vi "Get 2D Array Double.vi"(5 "use temporary file? (F)":bool, 7 "data type of variable":dbl[][](array[numeric]), 8 "error in":errorcluster, 10 "variable name":string, 11 "GOLPI ref. in":T1={"pipe handle"={"lv_proc.dll file path"=path "", "process instance handle"=[], "debug mode"=FALSE, "debug data"=[]}, "fast read timeout [ms]"=500, "fast read settle time [ms]"=10, "fast read to multiple [ms]"=1, "max elements per input line"=100, "slow read timeout [ms]"=5000, "stdin double format specifier"="%_16e", "max elements per stdout output column"=100, "console mode bitstream"=FALSE, "bitstream first read timeout [ms]"=1000, "bitstream read timeout [ms]"=50, "struct transfer possible"=FALSE, "matlab mode"=FALSE}) -> (0 "error out":errorcluster, 2 "value":dbl[][](array[numeric]) format="%.2f", 3 "GOLPI ref. out":T1={"pipe handle"={"lv_proc.dll file path"=path "", "process instance handle"=[], "debug mode"=FALSE, "debug data"=[]}, "fast read timeout [ms]"=500, "fast read settle time [ms]"=10, "fast read to multiple [ms]"=1, "max elements per input line"=100, "slow read timeout [ms]"=5000, "stdin double format specifier"="%_16e", "max elements per stdout output column"=100, "console mode bitstream"=FALSE, "bitstream first read timeout [ms]"=1000, "bitstream read timeout [ms]"=50, "struct transfer possible"=FALSE, "matlab mode"=FALSE})   [LabVIEW 2020, in "GOLPI library.lvlib"]
doc: "Part of polymorph Get Variable.vi"
uses:
  GOLPI library.lvlib
  GOLPI reference Type Def.ctl
  Pipe Handle.ctl
  Bitstream Data Type.ctl
  Custom Error Codes Enum Type Def.vi
  LV Process library.lvlib
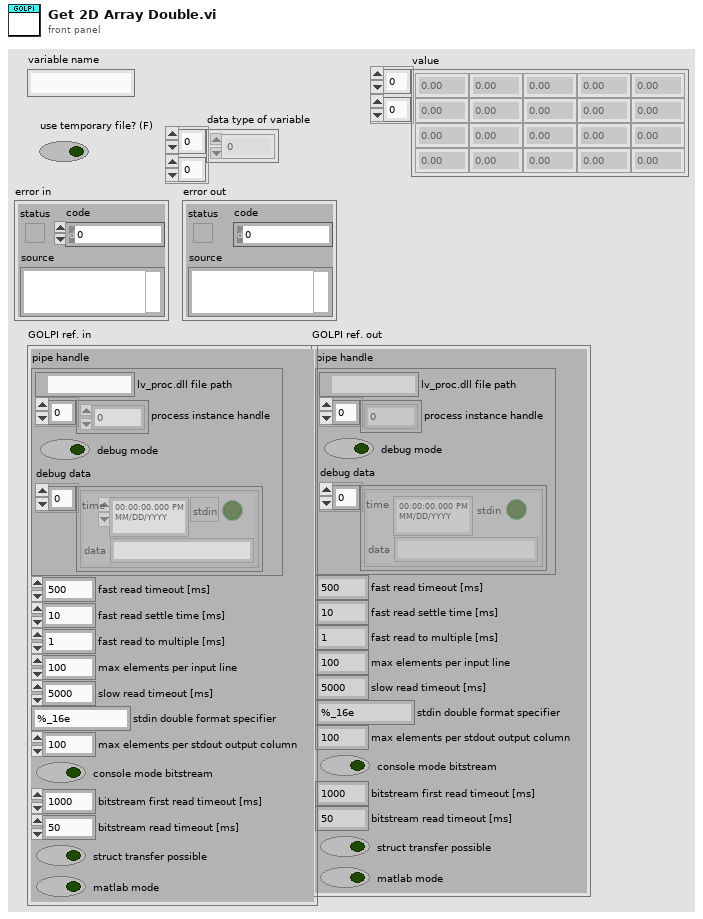
[diagram p1: front panel]
types:
  T1 = typedef "GOLPI library.lvlib/GOLPI reference Type Def.ctl" = cluster{"pipe handle":T2, "fast read timeout [ms]":u32, "fast read settle time [ms]":u32, "fast read to multiple [ms]":u32, "max elements per input line":u32, "slow read timeout [ms]":u32, "stdin double format specifier":string, "max elements per stdout output column":u32, "console mode bitstream":bool, "bitstream first read timeout [ms]":u32, "bitstream read timeout [ms]":u32, "struct transfer possible":bool, "matlab mode":bool}
  T2 = typedef "LV Process library.lvlib/Pipe Handle.ctl" = cluster{"lv_proc.dll file path":path, "process instance handle":u32[], "debug mode":bool, "debug data":cluster{"time":timestamp, "stdin":bool, "data":string}[]}
  T3 = typedef "GOLPI library.lvlib/Bitstream Data Type.ctl" = enum16{"dummy", "int", "uint", "float", "complex", "str", "real numeric"}
  T4 = typedef "GOLPI library.lvlib/Custom Error Codes Enum Type Def.vi" = enum16{"no error", "00 working directory PAR1 missing", "01 octave binary PAR1 missing", "02 octave report error PAR1", "03 empty output last cmd PAR1", "04 missing temporary file PAR1", "05 pwd PAR 1 not exist", "06 oct package not installed", "07 octave default binary missing", "10 var PAR1 not string, vect", "11 var PAR1 not num, scal, ~compl", "12 var PAR1 not num, scal, compl", "13 var PAR1 not num, vect, ~compl", "14 var PAR1 not num, vect, compl", "15 var PAR1 not num, mat, ~compl", "16 var PAR1 not num, mat, ~compl", "30 read timeout", "60 bitstream transport failed", "61 bitstream decode error PAR1", "62 bitstream cannot be set", "70 struct transfer not possible", "80 struct: cluster elem. PAR1 not implem.", "81 struct: structure field PAR1 not implem.", "82 struct: size mismatch of PAR1", "83 struct: type mismatch of PAR1", "98 internal error", "99 not finished", "90 Not supported in Matlab mode", "91 Matlab variable transfer error", "92 Matlab Script Error"}
  T5 = typedef "GOLPI library.lvlib/Bitstream Data.ctl" = cluster{"double":dbl[][], "cplx double":cdb[][], "int64":i64[][], "uint64":u64[][], "str":string[], "data type":T3}
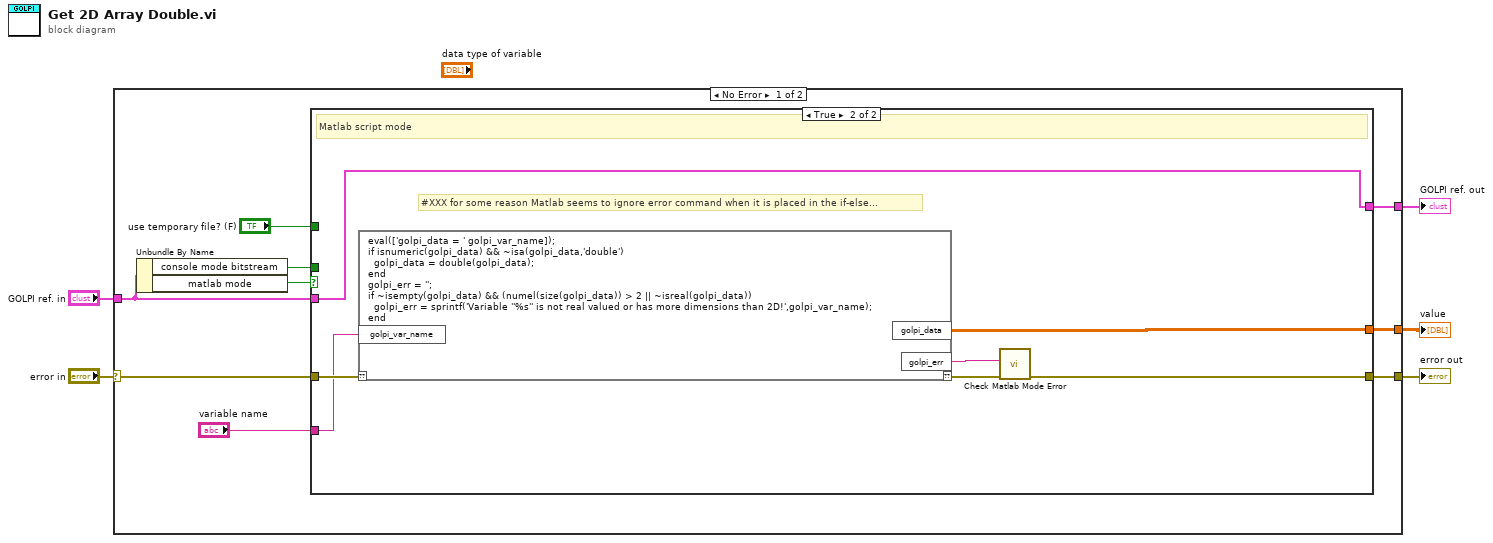
[diagram p0: block diagram]
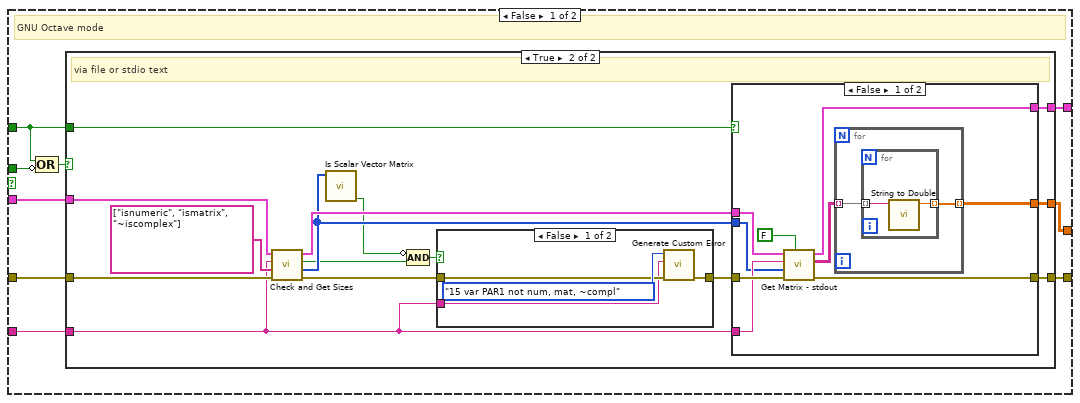
[diagram p2: hidden frame]
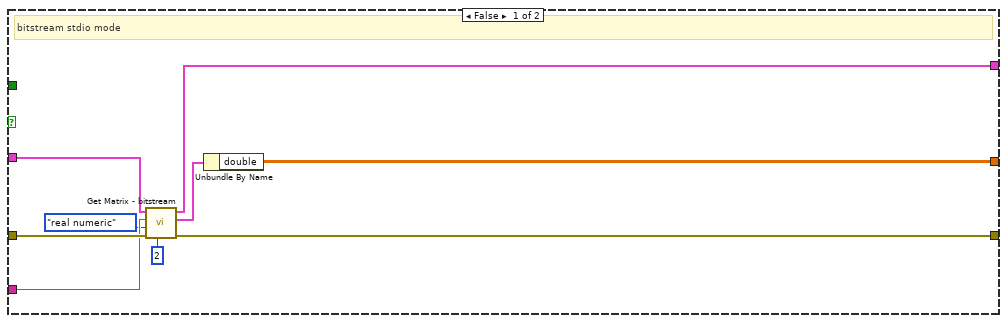
[diagram p3: hidden frame]
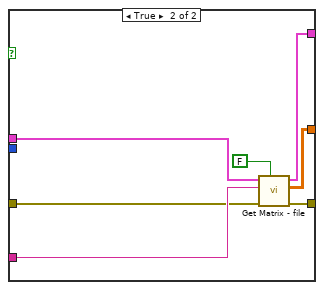
[diagram p4: hidden frame]
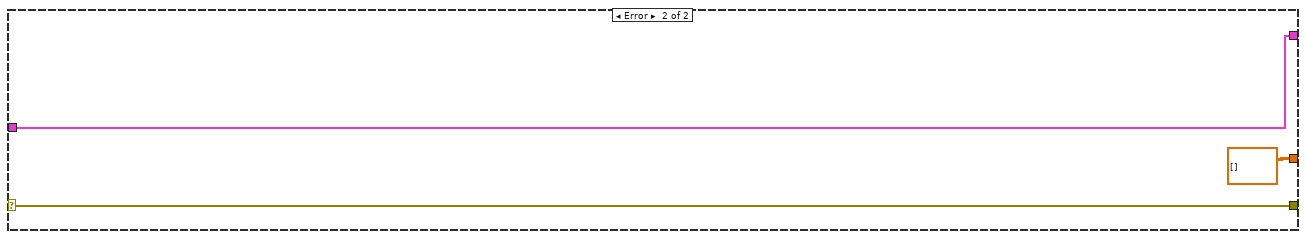
[diagram p6: hidden frame]
diagram:
  n1 = case shown="No Error" "error in" {
    selector: "error in" -> [w13 w82]
    tunnel: [w12 w82] -> w5
    tunnel: [w14 dbl[][] [] ("double array")] -> w3
    tunnel: "GOLPI ref. in" -> [w9 w80]
    tunnel: [w10 w80] -> w1
    frame No Error {
      n2 = Unbundle By Name(w9) -> ("console mode bitstream"=w8:bool, "matlab mode"=w6:bool)
      n3 = case shown="True" w6 {
        tunnel: [w23 w76] -> w14
        tunnel: w13 -> [w22 w79]
        tunnel: [w21 w73] -> w12
        tunnel: "variable name" -> [w20 w78]
        tunnel: [w19 w77] -> w10
        tunnel: w9 -> [w18 w77]
        tunnel: w8 -> [w17 _]
        tunnel: "use temporary file? (F)" -> [w16 _]
        frame False {
          # "GNU Octave mode"
          n4 = Compound Arithmetic op=OR(w16, invert w17) -> (w15:bool)
          n5 = case shown="True" w15 {
            tunnel: [w24 w47] -> w23
            tunnel: w22 -> [w32 w46]
            tunnel: [w27 w41] -> w21
            tunnel: w20 -> [w30 w40]
            tunnel: [w26 w39] -> w19
            tunnel: w18 -> [w31 w34]
            tunnel: w16 -> [_ w33]
            frame False {
              # "bitstream stdio mode"
              n6 = call "Get Matrix - bitstream.vi"("max dimensions (0: scalar)"=2, "error in (no error)"=w32, "data type"=Bitstream_Data_Type."real numeric", "variable name"=w30, "GOLPI ref. in"=w31) -> ("error out"=w27:errorcluster, "data"=w25:T5, "GOLPI ref. out"=w26:T1)  [unwired: 4 in]
              n7 = Unbundle By Name(w25) -> ("double"=w24:dbl[][])
            }
            frame True {
              # "via file or stdio text"
              n8 = call "Check and Get Sizes.vi"("error in (no error)"=w46, "test commands"=string[] ["isnumeric", "ismatrix", "~iscomplex"], "variable name"=w40, "GOLPI ref. in"=w34) -> ("error out"=w45:errorcluster, "octave sizes"=w38:i32[], "all tests OK?"=w36:bool, "GOLPI ref. out"=w43:T1)  [unwired: 4 in]
              n9 = call "Is Scalar Vector Matrix.vi"("octave sizes"=w38) -> ("is >2d matrix?"=w35:bool)  [unwired: 5 in, 5 out]
              n10 = Compound Arithmetic op=AND(invert w35, w36) -> (w37:bool)
              n11 = case shown="False" w37 {
                tunnel: w45 -> [w70 w72]
                tunnel: [w69 w72] -> w42
                tunnel: w40 -> [w68 _]
                frame False {
                  n12 = call "Generate Custom Error.vi"("error in"=w70, "PAR1"=w68, "GOLPI error"=Custom_Error_Codes_Enum_Type_Def.vi."15 var PAR1 not num, mat, ~compl" ("Enum")) -> ("error out"=w69:errorcluster)  [unwired: 8 in]
                }
                frame True {
                }
              }
              n13 = case shown="False" w33 {
                tunnel: [w48 w61] -> w47
                tunnel: w43 -> [w53 w66]
                tunnel: [w50 w65] -> w39
                tunnel: w42 -> [w56 w63]
                tunnel: [w55 w62] -> w41
                tunnel: w40 -> [w54 w64]
                tunnel: w38 -> [w51 _]
                frame False {
                  n14 = call "Get Matrix - stdout.vi"("is string?"=FALSE ("is string"), "error in (no error)"=w56, "octave sizes"=w51, "variable name"=w54, "GOLPI ref. in"=w53) -> ("error out"=w55:errorcluster, "array"=w49:string[][], "GOLPI ref. out"=w50:T1)  [unwired: 4 in]
                  n15 = for {
                    tunnel: w49 -> [w58] mode=indexing
                    tunnel: [w57] -> w48 mode=indexing
                    n16 = for {
                      tunnel: w58 -> [w60] mode=indexing
                      tunnel: [w59] -> w57 mode=indexing
                      n17 = call "String to Double.vi"("string"=w60) -> ("number"=w59:dbl)  [unwired: 10 in]
                    }
                  }
                }
                frame True {
                  n18 = call "Get Matrix - file.vi"("is string?"=FALSE ("is string"), "error in (no error)"=w63, "variable name"=w64, "GOLPI ref. in"=w66) -> ("error out"=w62:errorcluster, "double array"=w61:dbl[][], "GOLPI ref. out"=w65:T1)  [unwired: 3 in, 2 out]
                }
              }
            }
          }
        }
        frame True {
          # "#XXX for some reason Matlab seems to ignore error command when it is placed in the if-else..."
          # "Matlab script mode"
          n19 = script code="eval(['golpi_data = ' golpi_var_name]);\nif isnumeric(golpi_data) && ~isa(golpi_data,'double')\n  golpi_data = double(golpi_data);\nend\ngolpi_err = '';\nif ~isempty(golpi_data) && (numel(size(golpi_data)) > 2 || ~isreal(golpi_data))\n  golpi_err = sprintf('Variable ''%s'' is not real valued or has more dimensions than 2D!',golpi_var_name);\nend"("??"=w79, "golpi_var_name"=w78) -> ("??"=w75:errorcluster, "golpi_data"=w76:dbl[][], "golpi_err"=w74:string)
          n20 = call "Check Matlab Mode Error.vi"("error in"=w75, "custom error string (empty)"=w74) -> ("error out"=w73:errorcluster)  [unwired: 9 in]
        }
      }
    }
    frame Error {
    }
  }
  "value" <- w3
  "error out" <- w5
  "GOLPI ref. out" <- w1
